vi "thcd_400_main.vi"(7 "stop_external":refnum<vi>, 8 "variable_ref":T1) -> ()   [LabVIEW 2019]
uses:
  thcd_controls/ctrl_chn_thcd.ctl
  thcd_controls/variable_reference.ctl
  thcd_controls/ctrl_sms_thcd.ctl
  <vilib>/Analysis/baseanly.llb/Mean (DBL).vi
  thcd_commands/thcd_set_samp.vi
  thcd_commands/thcd_get_samp.vi
  <vilib>/Analysis/NI_AALBase.lvlib
panel:
  in  "n_avg":i32
  out "current_point_ch2":dbl caption="Current Point"
  out "current_point_ch1":dbl caption="Current Point"
  in  "close_ch2":bool
  in  "open_ch2":bool
  in  "close":bool
  in  "open":bool
  out "status_log":bool caption="Status"
  in  "Logging":bool=TRUE
  out "thcd_st_ch2":bool caption="Status"
  out "thcd_res_msg_ch2":string caption="Msg"
  in  "thcd_val_ch2":dbl=0.1 caption="Set Point" min=0.1 max=10000.0 format="%#.6g"
  in  "set_ch2":bool
  out "Last Updated":timestamp format="%<%Y-%m-%d %H:%M:%S>T"
  out "Sensor data":cluster{cluster{"X":dbl, "Y":dbl}[]}[](graph)
  out "thcd_st":bool caption="Status"
  out "thcd_res_msg":string caption="Msg"
  in  "thcd_val":dbl=0.1 caption="Set Point" min=0.1 max=10000.0 format="%#_5f"
  in  "wait_sec":u32=1000 caption="Interval (s)"
  out "thcd_res_4":T3
  out "thcd_res_3":T3
  out "thcd_res_2":T3
  out "thcd_res_1":T3
  in  "getstat":bool
  in  "set":bool
  in  "read":bool
  out "FM1":dbl caption="L/m" format="%.2f"
  out "FC2":dbl caption="L/m" format="%.2f"
  out "FC1":dbl caption="L/m" format="%.2f"
  in  "Baud_rate":u32(ring)=9600 items=["9.6KHz"=9600, "19.2KHz"=19200]
  in  "VISA":refnum<visa-resource-name>="COM13"
  in  "Init Devices":bool
  in  "Exit":bool
  # "THCD-400 :  Mass Flow Controll & Monitor"
  # "Flow Control: FC1 (Ch 1)"
  # "Flow Control: FC2 (Ch 2)"
  # "Magnet Flow:"
  # "Separator Flow:"
  # "Fridge Flow:"
  # "Set Range:\n0.1-10000"
  # "\"res_state\" must be \"CLOSE\" (which actually means \"AUTO\") to control the flow rates remotely.  If it is not, change it by using the hardware button of THCD-400."
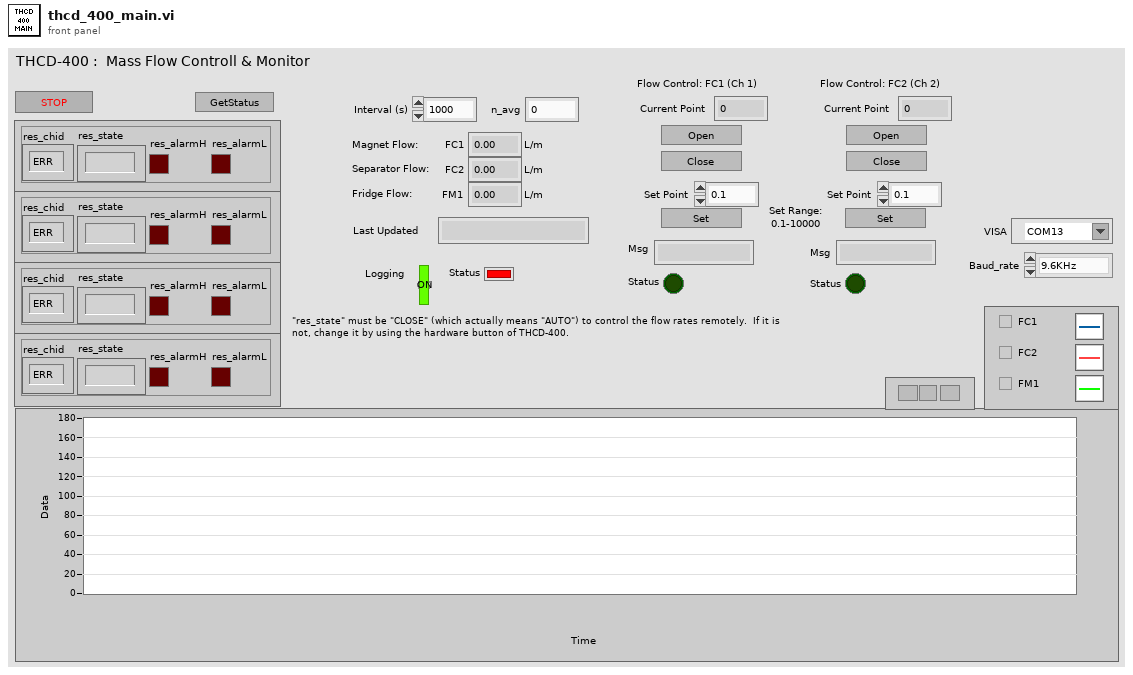
[diagram p1: front panel]
types:
  T1 = typedef "variable_reference.ctl" = cluster{"Status":refnum<vi>, "FM1":refnum<vi>, "FC1":refnum<vi>, "FC2":refnum<vi>}
  T2 = typedef "ctrl_chn_thcd.ctl" = enum8{"ERR", "1", "2", "3", "4"}
  T3 = cluster{"res_chid":T2, "res_state":string, "res_alarmH":bool, "res_alarmL":bool}
  T4 = typedef "ctrl_sms_thcd.ctl" = enum16{"idle", "init", "exit", "read", "open", "close", "set", "open_ch2", "close_ch2", "set_ch2", "getstat"}
  T5 = enum16{"SetPoint", "AlarmH", "AlarmL", "Multiplier", "CalibValue"}
  T6 = cluster{"res_chid":T2, "res_val":dbl, "res_uom":string, "res_gid":string}[]
  T7 = cluster{"res_chid":T2, "res_val":dbl, "res_uom":string, "res_gid":string}
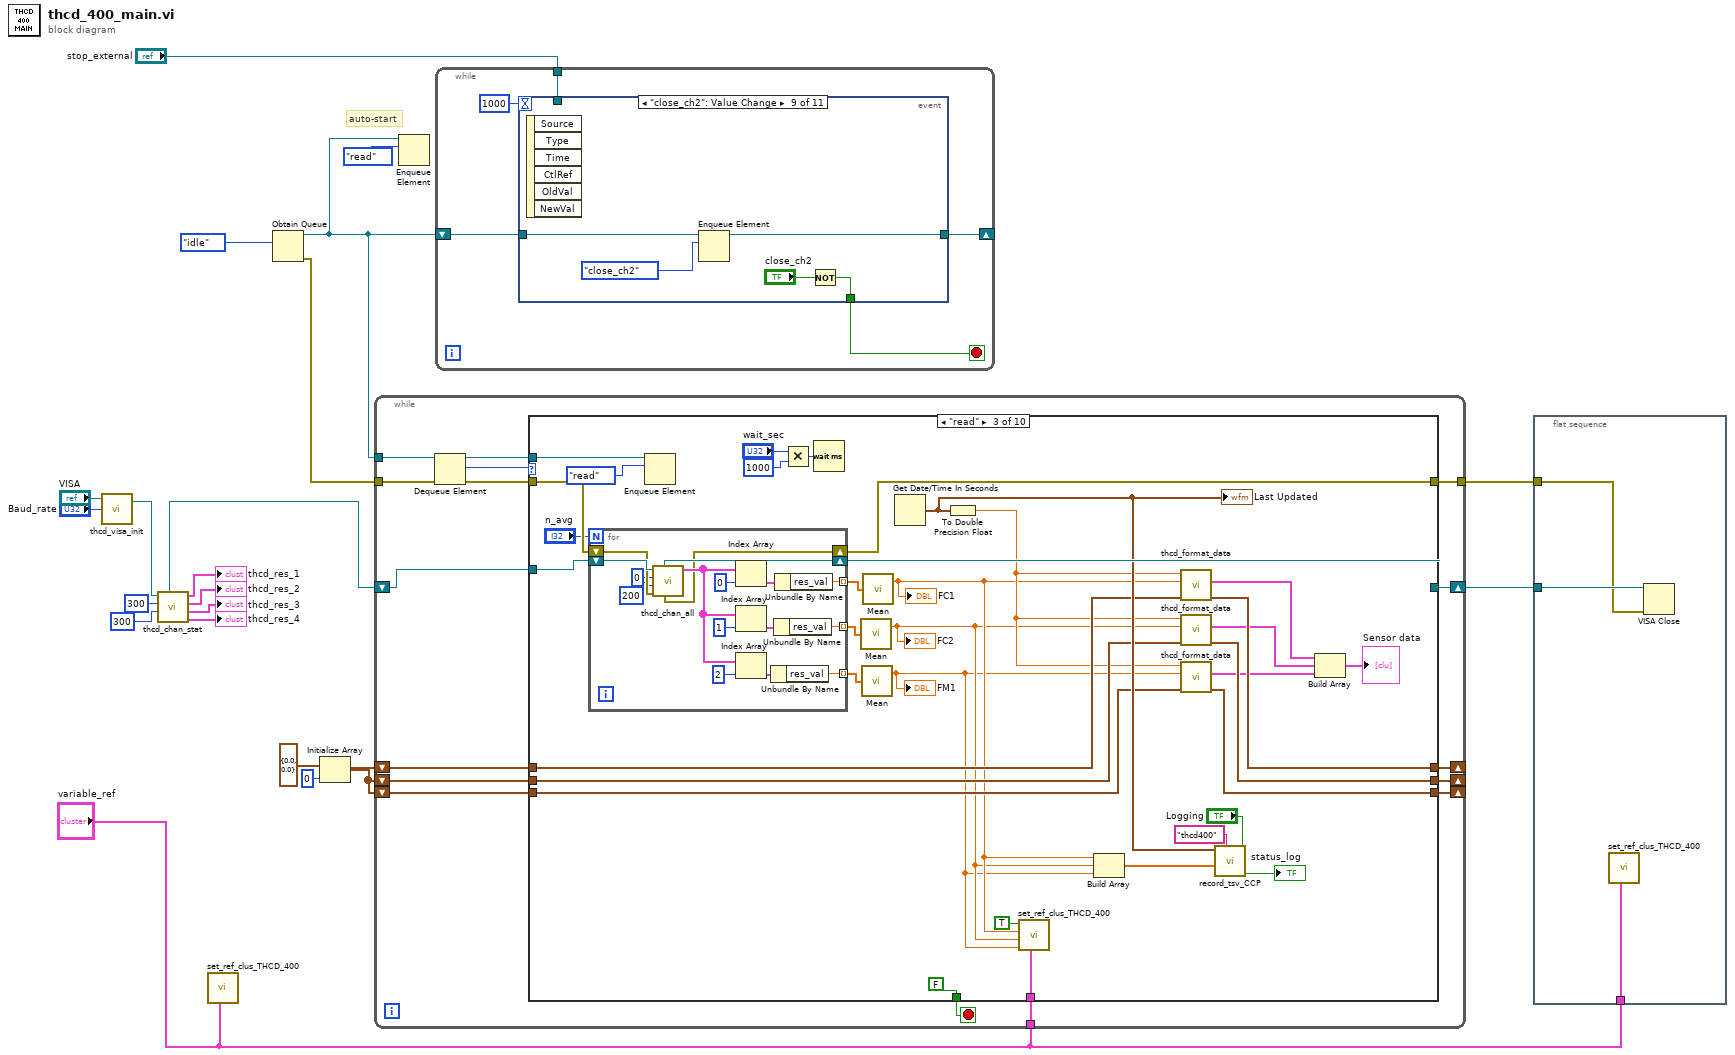
[diagram p0: block diagram]
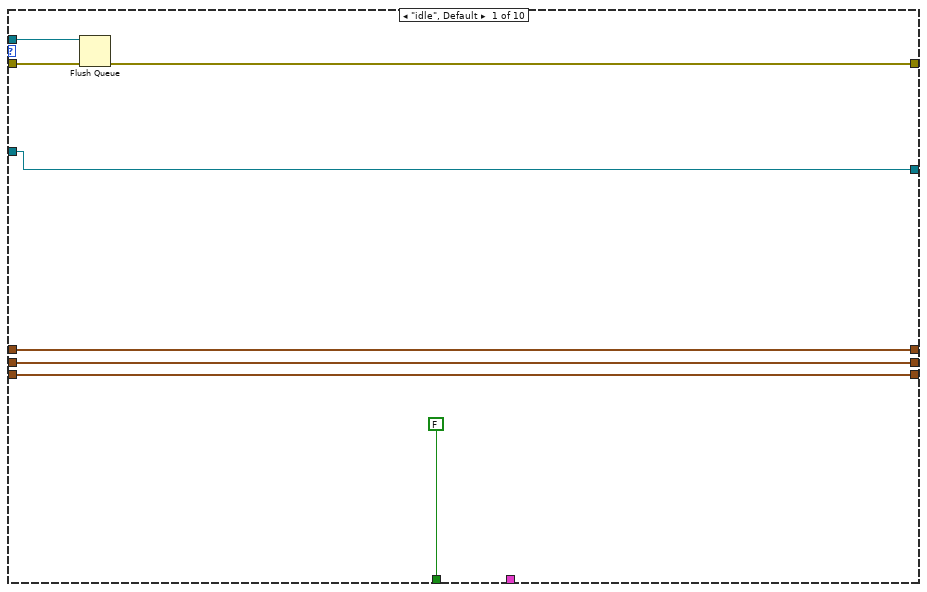
[diagram p2: hidden frame]
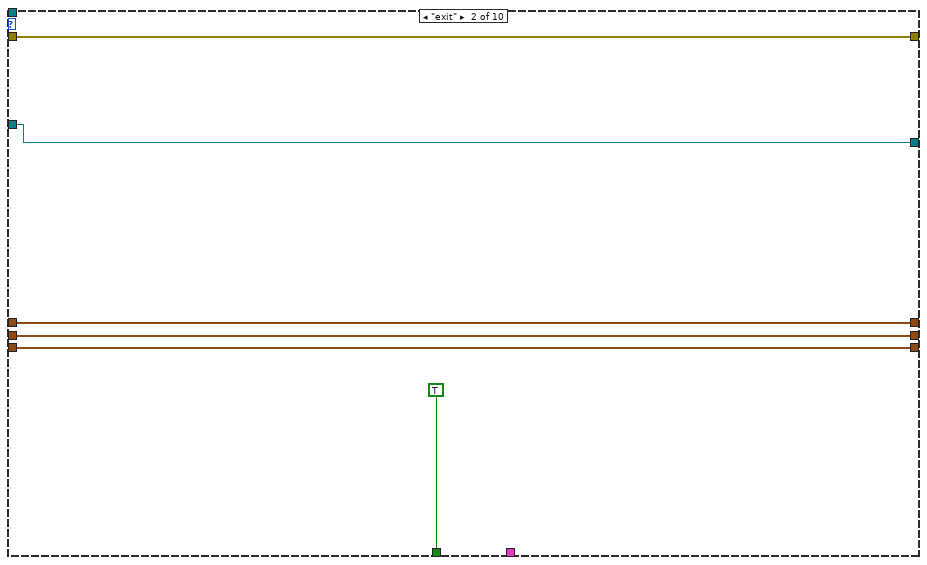
[diagram p3: hidden frame]
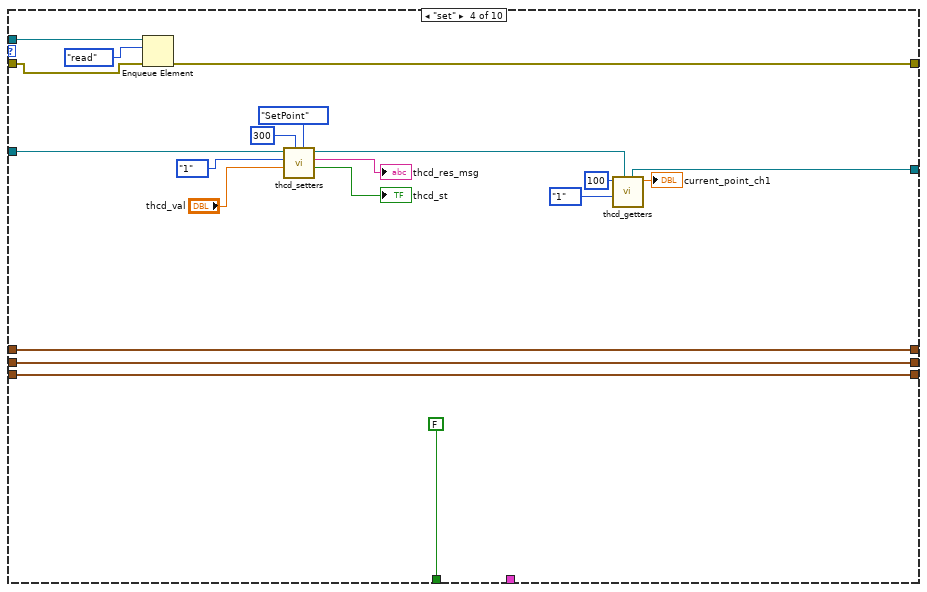
[diagram p4: hidden frame]
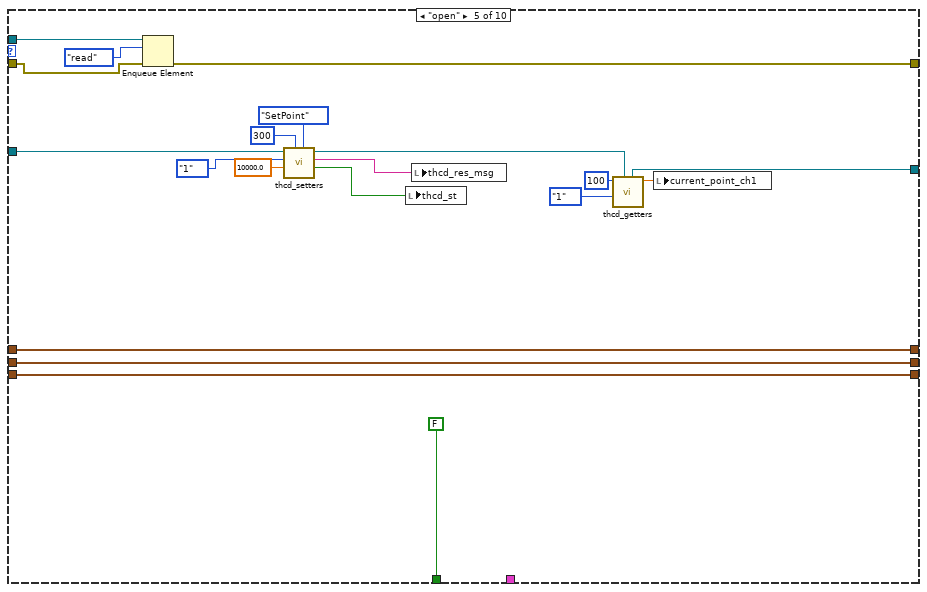
[diagram p5: hidden frame]
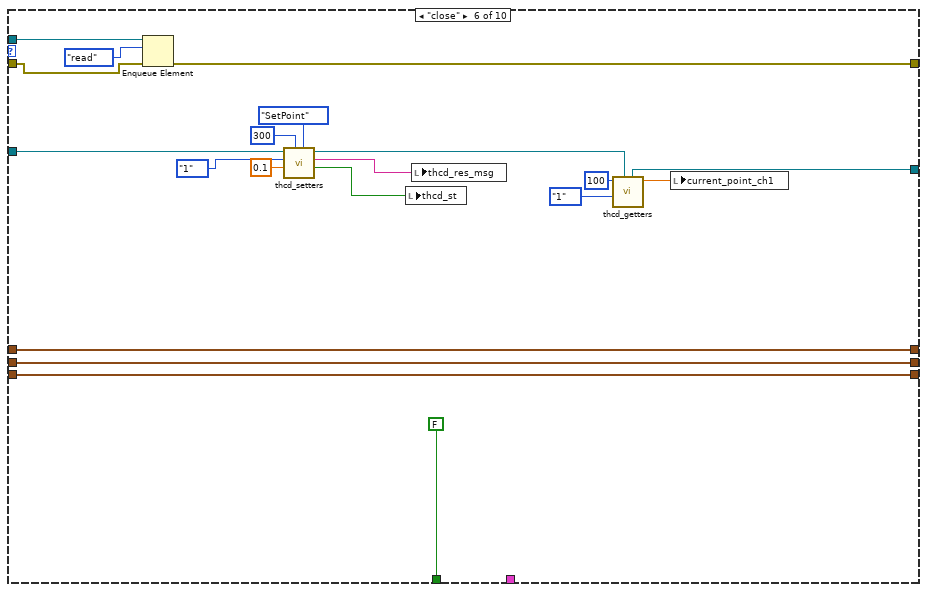
[diagram p6: hidden frame]
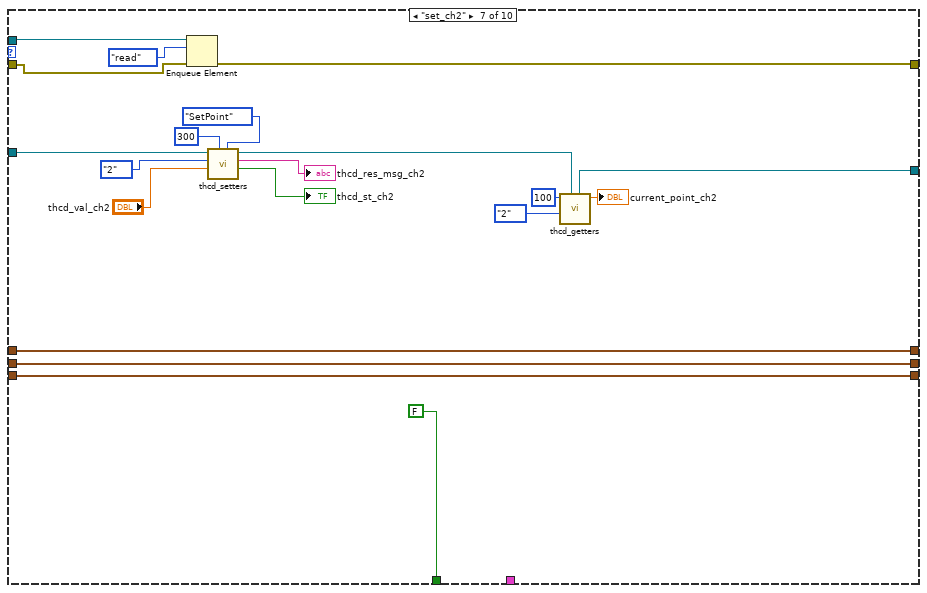
[diagram p7: hidden frame]
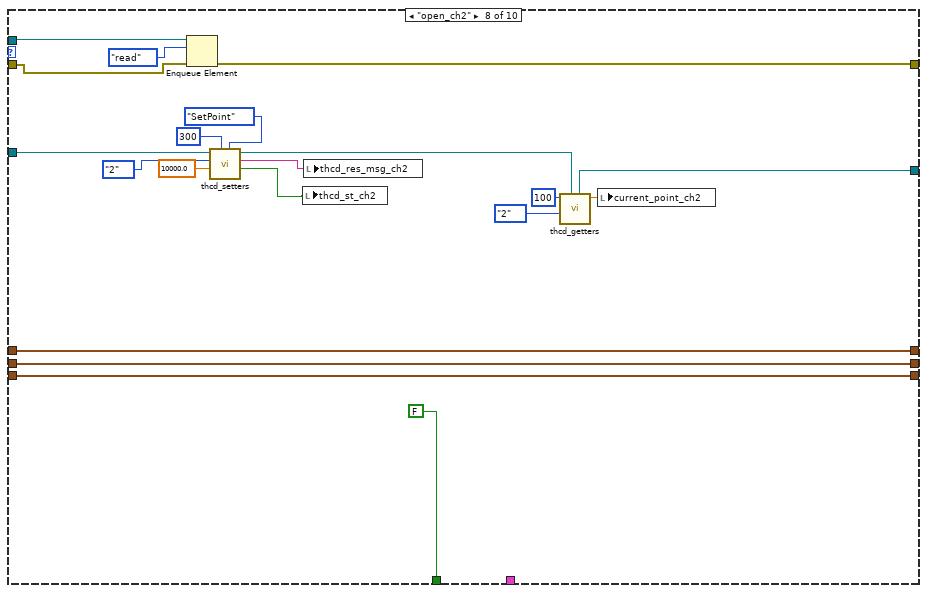
[diagram p8: hidden frame]
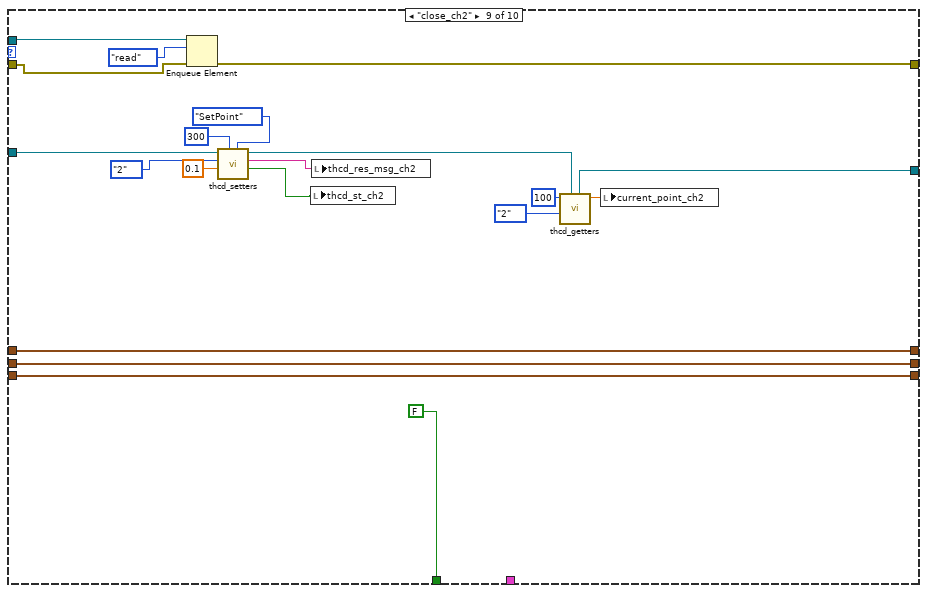
[diagram p9: hidden frame]
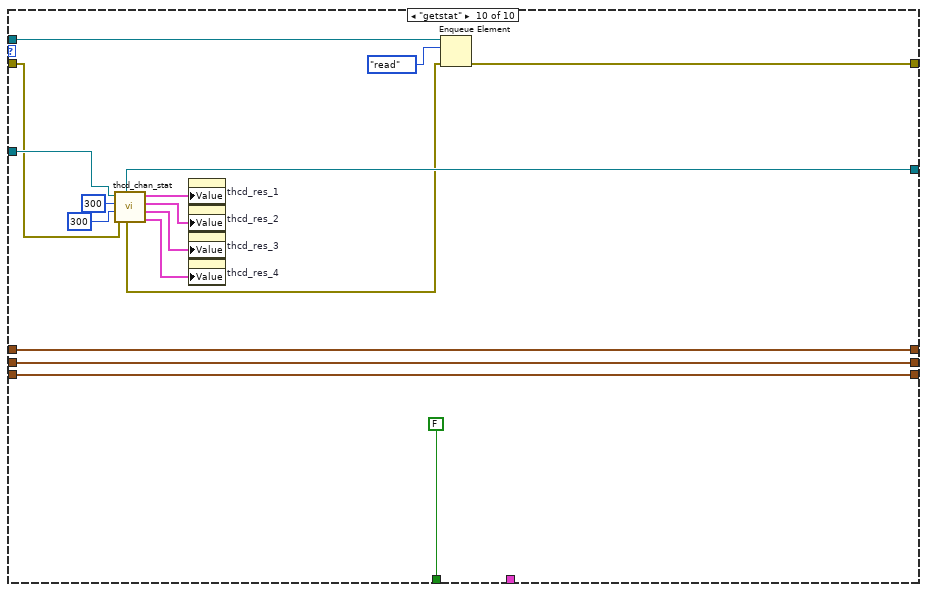
[diagram p10: hidden frame]
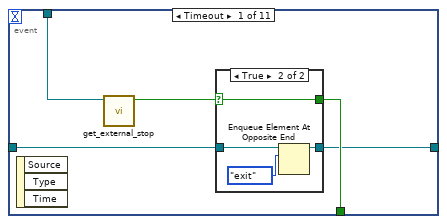
[diagram p11: hidden frame]
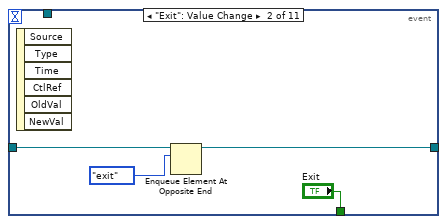
[diagram p13: hidden frame]
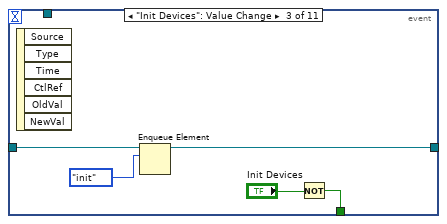
[diagram p14: hidden frame]
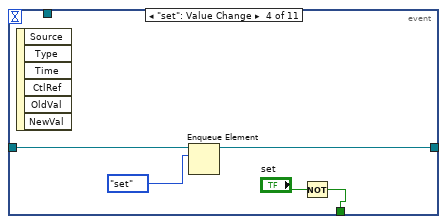
[diagram p15: hidden frame]
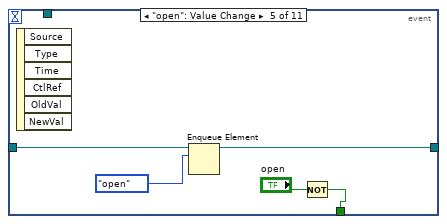
[diagram p16: hidden frame]
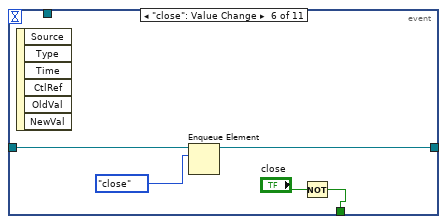
[diagram p17: hidden frame]
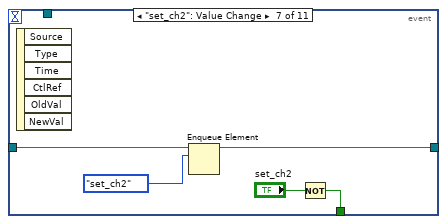
[diagram p18: hidden frame]
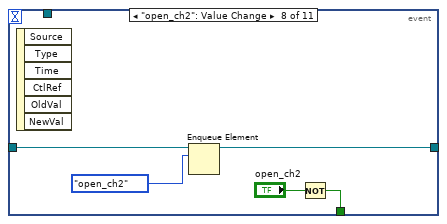
[diagram p19: hidden frame]
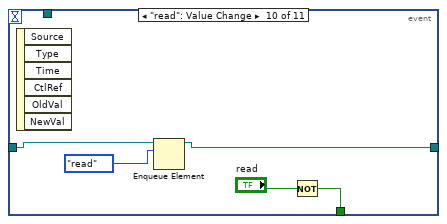
[diagram p20: hidden frame]
diagram:
  # "auto-start"
  n1 = call "thcd_visa_init.vi"("Serial Settings:Baud Rate"="Baud_rate", "thcd_visa"="VISA") -> ("thcd_visa"=w8:refnum<visa-resource-name>)  [unwired: 1 in, 1 out]
  n2 = call "thcd_chan_stat.vi"("thcd_b2r"=u32 300, "thcd_delay"=u32 300, "thcd_visa"=w8) -> ("thcd_res_4"=→"thcd_res_4":T3, "thcd_res_3"=→"thcd_res_3":T3, "thcd_res_2"=→"thcd_res_2":T3, "thcd_res_1"=→"thcd_res_1":T3, "thcd_visa"=w7:refnum<visa-resource-name>)  [unwired: 1 in, 3 out]
  n3 = call "set_ref_clus_THCD_400.vi"("variable_ref"="variable_ref") -> ()  [unwired: 11 in]
  n4 = Obtain Queue(element data type=ctrl_sms_thcd."idle" ("Enum")) -> (queue out=w5:refnum<queue>, error out=w20:errorcluster)  [unwired: 4 in, 1 out]
  n5 = Initialize Array(cluster{"X":dbl, "Y":dbl} {"X"=0.0, "Y"=0.0}, 0 ("dimension size")) -> (w17:cluster{"X":dbl, "Y":dbl}[])
  n6 = while {
    tunnel: w20 -> [w35]
    tunnel: [w32] -> w3
    tunnel: w5 -> [w36]
    shift-right: [w23] -> w4
    shift-left: w7 -> [w30]
    shift-right: [w26] -> _
    shift-left: w17 -> [w29]
    shift-right: [w25] -> _
    shift-left: w17 -> [w28]
    shift-right: [w24] -> _
    shift-left: w17 -> [w27]
    tunnel: "variable_ref" -> [w22]
    stop <- w37 stop-if-true
    n7 = Dequeue Element(queue=w36, error in (no error)=w35) -> (queue out=w31:refnum<queue>, element=w34:T4, error out=w33:errorcluster)  [unwired: 1 in, 1 out]
    n8 = case shown="\"read\"" w34 {
      tunnel: w31 -> [w44 _ w80 w120 w140 w160 w175 w198 w218 w238]
      tunnel: [FALSE TRUE FALSE FALSE FALSE FALSE FALSE FALSE FALSE FALSE] -> w37
      tunnel: w33 -> [w43 w50 w85 w119 w139 w159 w174 w197 w217 w224]
      tunnel: [w42 w50 w83 w118 w138 w158 w173 w196 w216 w237] -> w32
      tunnel: [w41 w49 w84 w106 w124 w144 w163 w184 w204 w229] -> w23
      tunnel: w30 -> [w41 w49 w86 w117 w137 w157 w172 w195 w215 w230]
      tunnel: w29 -> [w40 w48 w71 w110 w133 w153 w170 w193 w213 w235]
      tunnel: w28 -> [w39 w47 w68 w109 w132 w152 w169 w192 w212 w234]
      tunnel: w27 -> [w38 w46 w64 w108 w131 w151 w168 w191 w211 w233]
      tunnel: [w40 w48 w70 w110 w133 w153 w170 w193 w213 w235] -> w26
      tunnel: [w39 w47 w67 w109 w132 w152 w169 w192 w212 w234] -> w25
      tunnel: [w38 w46 w63 w108 w131 w151 w168 w191 w211 w233] -> w24
      tunnel: w22 -> [_ _ w78 _ _ _ _ _ _ _]
      frame "idle", Default {
        n9 = Flush Queue(queue=w44, error in (no error)=w43) -> (error out=w42:errorcluster)  [unwired: 2 out]
      }
      frame "exit" {
      }
      frame "read" {
        n10 = for {
          N: "n_avg" -> [_]
          tunnel: [w89] -> w60 mode=indexing
          tunnel: [w88] -> w56 mode=indexing
          tunnel: [w87] -> w55 mode=indexing
          shift-right: [w98] -> w84
          shift-left: w86 -> [w102]
          shift-right: [w90] -> w83
          shift-left: w85 -> [w101]
          n11 = call "thcd_chan_all.vi"("err_in"=w101, "thcd_b2r"=u32 200, "thcd_delay"=u32 0, "thcd_visa"=w102) -> ("thcd_res"=w91:T6, "err_out"=w90:errorcluster, "thcd_visa"=w98:refnum<visa-resource-name>)  [unwired: 3 in, 2 out]
          n12 = Index Array(array=w91, index=0) -> (element=w96:T7)
          n13 = Index Array(array=w91, index=1) -> (element=w95:T7)
          n14 = Index Array(array=w91, index=2) -> (element=w94:T7)
          n15 = Unbundle By Name(w94) -> ("res_val"=w87:dbl)
          n16 = Unbundle By Name(w95) -> ("res_val"=w88:dbl)
          n17 = Unbundle By Name(w96) -> ("res_val"=w89:dbl)
        }
        n18 = Enqueue Element(queue=w80, element=ctrl_sms_thcd."read") -> ()  [unwired: 2 in, 3 out]
        n19 = Multiply(x="wait_sec", y=u32 1000) -> (x*y=w54:u32)
        n20 = Wait (ms)(milliseconds to wait=w54) -> ()  [unwired: 1 out]
        n21 = call-poly <vilib>:"Mean.vi"("X"=w56) -> ("mean"=w58:dbl)  [unwired: 1 out]
        "FC2" <- w58
        n22 = call-poly <vilib>:"Mean.vi"("X"=w55) -> ("mean"=w57:dbl)  [unwired: 1 out]
        "FM1" <- w57
        n23 = call-poly <vilib>:"Mean.vi"("X"=w60) -> ("mean"=w59:dbl)  [unwired: 1 out]
        "FC1" <- w59
        n24 = Get Date/Time In Seconds() -> (seconds since 1Jan1904=w73:timestamp)
        "Last Updated" <- w73
        n25 = To Double Precision Float(number=w73) -> (double precision float=w65:dbl)
        n26 = call "set_ref_clus_THCD_400.vi"("variable_ref"=w78, "FM1"=w57, "FC2"=w58, "FC1"=w59, "status"=TRUE) -> ()  [unwired: 7 in]
        n27 = Build Array(w59, w58, w57) -> (w72:dbl[])
        n28 = call "thcd_format_data.vi"("array_in"=w71, "value"=w59, "time"=w65) -> ("array_out"=w70:cluster{"time":dbl, "value":dbl}[], "cluster_out"=w69:cluster{cluster{"time":dbl, "value":dbl}[]})  [unwired: 7 in]
        n29 = call "thcd_format_data.vi"("array_in"=w68, "value"=w58, "time"=w65) -> ("array_out"=w67:cluster{"time":dbl, "value":dbl}[], "cluster_out"=w66:cluster{cluster{"time":dbl, "value":dbl}[]})  [unwired: 7 in]
        n30 = call "thcd_format_data.vi"("array_in"=w64, "value"=w57, "time"=w65) -> ("array_out"=w63:cluster{"time":dbl, "value":dbl}[], "cluster_out"=w62:cluster{cluster{"time":dbl, "value":dbl}[]})  [unwired: 7 in]
        n31 = call "record_tsv_CCP.vi"("logging_on"="Logging", "folder_name"="thcd400", "value_array"=w72, "time"=w73) -> ("status"=→"status_log":bool)  [unwired: 6 in, 1 out]
        n32 = Build Array(w69, w66, w62) -> (→"Sensor data":cluster{cluster{"time":dbl, "value":dbl}[]}[])
      }
      frame "set" {
        n33 = Enqueue Element(queue=w120, element=ctrl_sms_thcd."read", error in (no error)=w119) -> (error out=w118:errorcluster)  [unwired: 1 in, 2 out]
        n34 = call-poly "thcd_setters.vi"("thcd_com"=T5."SetPoint", "thcd_delay"=u32 300, "thcd_val"="thcd_val", "thcd_ch"=ctrl_chn_thcd."1", "thcd_visa"=w117) -> ("thcd_st"=→"thcd_st":bool, "thcd_res_msg"=→"thcd_res_msg":string, "thcd_visa"=w107:refnum<visa-resource-name>)  [unwired: 1 in, 1 out]
        n35 = call-poly "thcd_getters.vi"("thcd_visa"=w107, "thcd_ch"=ctrl_chn_thcd."1", "thcd_delay"=u32 100) -> ("thcd_res"=→"current_point_ch1":dbl, "thcd_visa"=w106:refnum<visa-resource-name>)  [unwired: 3 in, 4 out]
      }
      frame "open" {
        n36 = Enqueue Element(queue=w140, element=ctrl_sms_thcd."read", error in (no error)=w139) -> (error out=w138:errorcluster)  [unwired: 1 in, 2 out]
        n37 = call-poly "thcd_setters.vi"("thcd_com"=T5."SetPoint", "thcd_delay"=u32 300, "thcd_val"=10000.0, "thcd_ch"=ctrl_chn_thcd."1", "thcd_visa"=w137) -> ("thcd_st"=w128:bool, "thcd_res_msg"=w129:string, "thcd_visa"=w125:refnum<visa-resource-name>)  [unwired: 1 in, 1 out]
        n38 = local write "thcd_st"(w128) -> ()
        n39 = local write "thcd_res_msg"(w129) -> ()
        n40 = call-poly "thcd_getters.vi"("thcd_visa"=w125, "thcd_ch"=ctrl_chn_thcd."1", "thcd_delay"=u32 100) -> ("thcd_res"=w123:dbl, "thcd_visa"=w124:refnum<visa-resource-name>)  [unwired: 3 in, 4 out]
        n41 = local write "current_point_ch1"(w123) -> ()
      }
      frame "close" {
        n42 = Enqueue Element(queue=w160, element=ctrl_sms_thcd."read", error in (no error)=w159) -> (error out=w158:errorcluster)  [unwired: 1 in, 2 out]
        n43 = call-poly "thcd_setters.vi"("thcd_com"=T5."SetPoint", "thcd_delay"=u32 300, "thcd_val"=0.1, "thcd_ch"=ctrl_chn_thcd."1", "thcd_visa"=w157) -> ("thcd_st"=w148:bool, "thcd_res_msg"=w149:string, "thcd_visa"=w145:refnum<visa-resource-name>)  [unwired: 1 in, 1 out]
        n44 = local write "thcd_st"(w148) -> ()
        n45 = local write "thcd_res_msg"(w149) -> ()
        n46 = call-poly "thcd_getters.vi"("thcd_visa"=w145, "thcd_ch"=ctrl_chn_thcd."1", "thcd_delay"=u32 100) -> ("thcd_res"=w143:dbl, "thcd_visa"=w144:refnum<visa-resource-name>)  [unwired: 3 in, 4 out]
        n47 = local write "current_point_ch1"(w143) -> ()
      }
      frame "set_ch2" {
        n48 = Enqueue Element(queue=w175, element=ctrl_sms_thcd."read", error in (no error)=w174) -> (error out=w173:errorcluster)  [unwired: 1 in, 2 out]
        n49 = call-poly "thcd_setters.vi"("thcd_com"=T5."SetPoint", "thcd_delay"=u32 300, "thcd_val"="thcd_val_ch2", "thcd_ch"=ctrl_chn_thcd."2", "thcd_visa"=w172) -> ("thcd_st"=→"thcd_st_ch2":bool, "thcd_res_msg"=→"thcd_res_msg_ch2":string, "thcd_visa"=w164:refnum<visa-resource-name>)  [unwired: 1 in, 1 out]
        n50 = call-poly "thcd_getters.vi"("thcd_visa"=w164, "thcd_ch"=ctrl_chn_thcd."2", "thcd_delay"=u32 100) -> ("thcd_res"=→"current_point_ch2":dbl, "thcd_visa"=w163:refnum<visa-resource-name>)  [unwired: 3 in, 4 out]
      }
      frame "open_ch2" {
        n51 = Enqueue Element(queue=w198, element=ctrl_sms_thcd."read", error in (no error)=w197) -> (error out=w196:errorcluster)  [unwired: 1 in, 2 out]
        n52 = call-poly "thcd_setters.vi"("thcd_com"=T5."SetPoint", "thcd_delay"=u32 300, "thcd_val"=10000.0, "thcd_ch"=ctrl_chn_thcd."2", "thcd_visa"=w195) -> ("thcd_st"=w188:bool, "thcd_res_msg"=w189:string, "thcd_visa"=w185:refnum<visa-resource-name>)  [unwired: 1 in, 1 out]
        n53 = local write "thcd_st_ch2"(w188) -> ()
        n54 = local write "thcd_res_msg_ch2"(w189) -> ()
        n55 = call-poly "thcd_getters.vi"("thcd_visa"=w185, "thcd_ch"=ctrl_chn_thcd."2", "thcd_delay"=u32 100) -> ("thcd_res"=w183:dbl, "thcd_visa"=w184:refnum<visa-resource-name>)  [unwired: 3 in, 4 out]
        n56 = local write "current_point_ch2"(w183) -> ()
      }
      frame "close_ch2" {
        n57 = Enqueue Element(queue=w218, element=ctrl_sms_thcd."read", error in (no error)=w217) -> (error out=w216:errorcluster)  [unwired: 1 in, 2 out]
        n58 = call-poly "thcd_setters.vi"("thcd_com"=T5."SetPoint", "thcd_delay"=u32 300, "thcd_val"=0.1, "thcd_ch"=ctrl_chn_thcd."2", "thcd_visa"=w215) -> ("thcd_st"=w208:bool, "thcd_res_msg"=w209:string, "thcd_visa"=w205:refnum<visa-resource-name>)  [unwired: 1 in, 1 out]
        n59 = local write "thcd_st_ch2"(w208) -> ()
        n60 = local write "thcd_res_msg_ch2"(w209) -> ()
        n61 = call-poly "thcd_getters.vi"("thcd_visa"=w205, "thcd_ch"=ctrl_chn_thcd."2", "thcd_delay"=u32 100) -> ("thcd_res"=w203:dbl, "thcd_visa"=w204:refnum<visa-resource-name>)  [unwired: 3 in, 4 out]
        n62 = local write "current_point_ch2"(w203) -> ()
      }
      frame "getstat" {
        n63 = call "thcd_chan_stat.vi"("err_in"=w224, "thcd_b2r"=u32 300, "thcd_delay"=u32 300, "thcd_visa"=w230) -> ("thcd_res_4"=w225:T3, "thcd_res_3"=w226:T3, "thcd_res_2"=w227:T3, "thcd_res_1"=w228:T3, "err_out"=w223:errorcluster, "thcd_visa"=w229:refnum<visa-resource-name>)  [unwired: 2 out]
        n64 = property on="thcd_res_1" class="Clust (strict)"("Value"=w228) -> ()  [unwired: 2 in, 2 out]
        n65 = property on="thcd_res_2" class="Clust (strict)"("Value"=w227) -> ()  [unwired: 2 in, 2 out]
        n66 = property on="thcd_res_3" class="Clust (strict)"("Value"=w226) -> ()  [unwired: 2 in, 2 out]
        n67 = property on="thcd_res_4" class="Clust (strict)"("Value"=w225) -> ()  [unwired: 2 in, 2 out]
        n68 = Enqueue Element(queue=w238, element=ctrl_sms_thcd."read", error in (no error)=w223) -> (error out=w237:errorcluster)  [unwired: 1 in, 2 out]
      }
    }
  }
  n69 = Enqueue Element(queue=w5, element=ctrl_sms_thcd."read") -> ()  [unwired: 2 in, 3 out]
  n70 = while {
    shift-right: [w243] -> _
    shift-left: w5 -> [w244]
    tunnel: "stop_external" -> [w241]
    stop <- w242 stop-if-true
    n71 = event shown="[8] \"close_ch2\": Value Change" {
      selector: _ -> [_ _ _ _ _ _ _ _ _ _ _]
      dyn-events: _ -> [_ _ _ _ _ _ _ _ _ _ _]
      timeout: 1000 -> [_ _ _ _ _ _ _ _ _ _ _]
      tunnel: w244 -> [w248 w259 w264 w266 w271 w276 w281 w286 w291 w297 w302]
      tunnel: [w247 w258 w263 w265 w270 w275 w280 w285 w290 w296 w301] -> w243
      tunnel: [w249 "Exit" w260 w268 w273 w278 w283 w288 w293 w298 w303] -> w242
      tunnel: w241 -> [w246 _ _ _ _ _ _ _ _ _ _]
      event Timeout {
        n72 = event-data() -> ()  [unwired: 1 in, 3 out]
        n73 = call "get_external_stop.vi"("ref_stop_external"=w246) -> ("stop_output"=w245:bool)  [unwired: 10 in]
        n74 = case shown="True" w245 {
          selector: w245 -> [w251 w255]
          tunnel: [w251 w255] -> w249
          tunnel: w248 -> [w250 w252]
          tunnel: [w250 w253] -> w247
          frame False {
          }
          frame True {
            n75 = Enqueue Element At Opposite End(queue=w252, element=ctrl_sms_thcd."exit" ("Enum")) -> (queue out=w253:refnum<queue>)  [unwired: 2 in, 2 out]
          }
        }
      }
      event "Exit": Value Change {
        n76 = event-data() -> ()  [unwired: 1 in, 6 out]
        n77 = Enqueue Element At Opposite End(queue=w259, element=ctrl_sms_thcd."exit" ("Enum")) -> (queue out=w258:refnum<queue>)  [unwired: 2 in, 2 out]
      }
      event "Init Devices": Value Change {
        n78 = event-data() -> ()  [unwired: 1 in, 6 out]
        n79 = Enqueue Element(queue=w264, element=ctrl_sms_thcd."init") -> (queue out=w263:refnum<queue>)  [unwired: 2 in, 2 out]
        n80 = Not(x="Init Devices") -> (.not. x?=w260:bool)
      }
      event "set": Value Change {
        n81 = event-data() -> ()  [unwired: 1 in, 6 out]
        n82 = Enqueue Element(queue=w266, element=ctrl_sms_thcd."set" ("Enum")) -> (queue out=w265:refnum<queue>)  [unwired: 2 in, 2 out]
        n83 = Not(x="set") -> (.not. x?=w268:bool)
      }
      event "open": Value Change {
        n84 = event-data() -> ()  [unwired: 1 in, 6 out]
        n85 = Enqueue Element(queue=w271, element=ctrl_sms_thcd."open" ("Enum")) -> (queue out=w270:refnum<queue>)  [unwired: 2 in, 2 out]
        n86 = Not(x="open") -> (.not. x?=w273:bool)
      }
      event "close": Value Change {
        n87 = event-data() -> ()  [unwired: 1 in, 6 out]
        n88 = Enqueue Element(queue=w276, element=ctrl_sms_thcd."close" ("Enum")) -> (queue out=w275:refnum<queue>)  [unwired: 2 in, 2 out]
        n89 = Not(x="close") -> (.not. x?=w278:bool)
      }
      event "set_ch2": Value Change {
        n90 = event-data() -> ()  [unwired: 1 in, 6 out]
        n91 = Enqueue Element(queue=w281, element=ctrl_sms_thcd."set_ch2" ("Enum")) -> (queue out=w280:refnum<queue>)  [unwired: 2 in, 2 out]
        n92 = Not(x="set_ch2") -> (.not. x?=w283:bool)
      }
      event "open_ch2": Value Change {
        n93 = event-data() -> ()  [unwired: 1 in, 6 out]
        n94 = Enqueue Element(queue=w286, element=ctrl_sms_thcd."open_ch2" ("Enum")) -> (queue out=w285:refnum<queue>)  [unwired: 2 in, 2 out]
        n95 = Not(x="open_ch2") -> (.not. x?=w288:bool)
      }
      event "close_ch2": Value Change {
        n96 = event-data() -> ()  [unwired: 1 in, 6 out]
        n97 = Enqueue Element(queue=w291, element=ctrl_sms_thcd."close_ch2" ("Enum")) -> (queue out=w290:refnum<queue>)  [unwired: 2 in, 2 out]
        n98 = Not(x="close_ch2") -> (.not. x?=w293:bool)
      }
      event "read": Value Change {
        n99 = event-data() -> ()  [unwired: 1 in, 6 out]
        n100 = Enqueue Element(queue=w297, element=ctrl_sms_thcd."read" ("Enum")) -> (queue out=w296:refnum<queue>)  [unwired: 2 in, 2 out]
        n101 = Not(x="read") -> (.not. x?=w298:bool)
      }
      event "getstat": Value Change {
        n102 = event-data() -> ()  [unwired: 1 in, 6 out]
        n103 = Enqueue Element(queue=w302, element=ctrl_sms_thcd."getstat") -> (queue out=w301:refnum<queue>)  [unwired: 2 in, 2 out]
        n104 = Not(x="getstat") -> (.not. x?=w303:bool)
      }
    }
  }
  n105 = flat-sequence {
    tunnel: w4 -> [w307]
    tunnel: w3 -> [w306]
    tunnel: "variable_ref" -> [w305]
    frame #0 {
      n106 = call "set_ref_clus_THCD_400.vi"("variable_ref"=w305) -> ()  [unwired: 11 in]
      n107 = VISA Close(VISA resource name=w307, error in (no error)=w306) -> ()  [unwired: 1 out]
    }
  }
